vi "MatchEndedDetector.vi"(8 "error in (no error)":errorcluster) -> (0 "error out":errorcluster, 3 "Match Ended":bool)   [LabVIEW 2018]
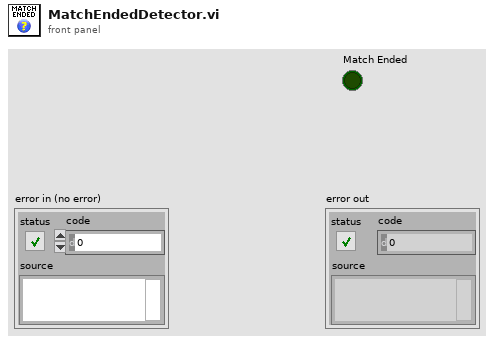
[diagram p1: front panel]
types:
  T1 = typedef "WPI_DriverStationRobotMode2.ctl" = enum16{"Autonomous Disabled", "Autonomous Enabled", "Teleop Disabled", "Teleop Enabled", "Disconnected", "Finish", "Test Disabled", "Test Enabled", "Emergency Stopped"}
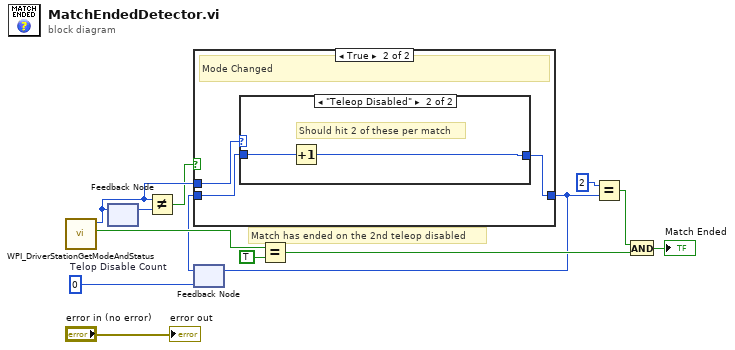
[diagram p0: block diagram]
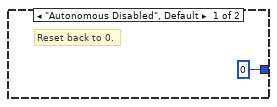
[diagram p3: hidden frame]
diagram:
  w5 = 0  # Telop Disable Count
  # "Match has ended on the 2nd teleop disabled"
  n1 = call <vilib>:"WPI_DriverStationGetModeAndStatus.vi"() -> ("FMS Attached"=w11:bool, "Robot Mode"=w7:T1)  [unwired: 10 in]
  n2 = feedback-in #1(w7) -> ()
  n3 = feedback #1() -> (w8:T1)  [unwired: 1 in]
  n4 = Not Equal?(x=w7, y=w8) -> (x != y?=w6:bool)
  n5 = feedback #2(w5) -> (w4:i32)
  n6 = case shown="True" w6 {
    tunnel: w7 -> [_ w17]
    tunnel: w4 -> [w14 w16]
    tunnel: [w14 w15] -> w1
    frame False {
      # "Mode hasn't changed, keep previous states"
    }
    frame True {
      # "Mode Changed"
      n7 = case shown="\"Teleop Disabled\"" w17 {
        tunnel: w16 -> [_ w20]
        tunnel: [0 w19] -> w15
        frame "Autonomous Disabled", Default {
          # "Reset back to 0."
        }
        frame "Teleop Disabled" {
          # "Should hit 2 of these per match"
          n8 = Increment(x=w20) -> (x+1=w19:i32)
        }
      }
    }
  }
  n9 = feedback-in #2(w1) -> ()
  n10 = Equal?(x=w11, y=TRUE) -> (x = y?=w13:bool)
  n11 = Equal?(x=2, y=w1) -> (x = y?=w2:bool)
  n12 = And(x=w2, y=w13) -> (x .and. y?=→"Match Ended":bool)
  "error out" <- "error in (no error)"
